vi "ivPIDantiWindup.vi"(4 "Saturation U":dbl, 6 "Saturation M":dbl, 7 "Reset":bool, 8 "PID Gains":cluster{"Kp":dbl, "Kd":dbl, "Ki":dbl, "Ts":dbl}={"Kp"=0.0, "Kd"=0.0, "Ki"=0.0, "Ts"=1.0}, 10 "Feedback":dbl, 11 "Reference":dbl) -> (3 "Control":dbl)   [LabVIEW 2016]
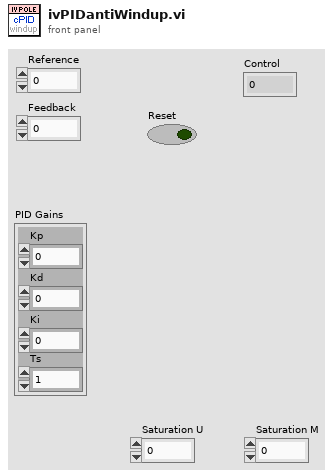
[diagram p1: front panel]
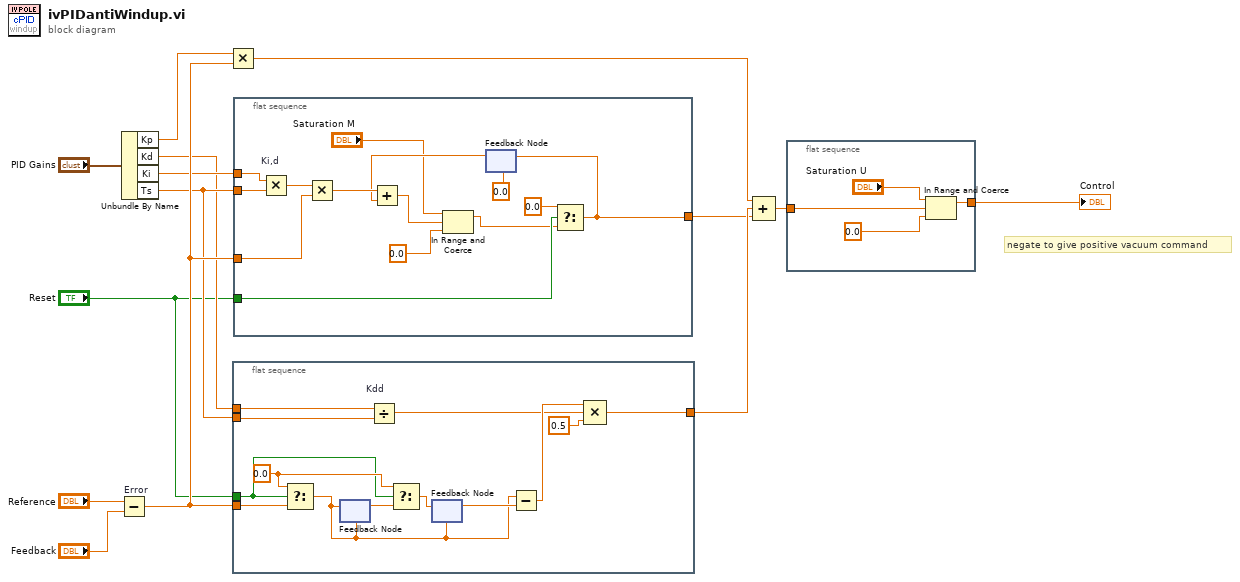
[diagram p0: block diagram]
diagram:
  # "negate to give positive vacuum command"
  n1 = Subtract "Error"(x="Reference", y="Feedback") -> (x-y=w7:dbl)
  n2 = Unbundle By Name("PID Gains") -> ("Kp"=w11:dbl, "Kd"=w4:dbl, "Ki"=w6:dbl, "Ts"=w5:dbl)
  n3 = Multiply(x=w11, y=w7) -> (x*y=w10:dbl)
  n4 = flat-sequence {
    tunnel: [w24] -> w9
    tunnel: w7 -> [w19]
    tunnel: w5 -> [w23]
    tunnel: w4 -> [w22]
    tunnel: "Reset" -> [w15]
    frame #0 {
      w16 = 0.0 ("t")
      n5 = Select(t=w16, s=w15, f=w19) -> (s? t:f=w20:dbl)
      n6 = feedback #1(w20) -> (w18:dbl)
      n7 = feedback-in #1(w20) -> ()
      n8 = Divide "Kdd"(x=w22, y=w23) -> (x/y=w21:dbl)
      n9 = Select(t=w16, s=w15, f=w18) -> (s? t:f=w17:dbl)
      n10 = feedback #2(w20) -> (w27:dbl)
      n11 = feedback-in #2(w17) -> ()
      n12 = Subtract(x=w20, y=w27) -> (x-y=w26:dbl)
      n13 = Compound Arithmetic op=MULTIPLY(w26, w21, 0.5 ("value")) -> (w24:dbl)
    }
  }
  n14 = flat-sequence {
    tunnel: [w30] -> w8
    tunnel: w7 -> [w41]
    tunnel: w6 -> [w39]
    tunnel: w5 -> [w37]
    tunnel: "Reset" -> [w33]
    frame #0 {
      n15 = Multiply "Ki,d"(x=w39, y=w37) -> (x*y=w38:dbl)
      n16 = Multiply(x=w38, y=w41) -> (x*y=w40:dbl)
      n17 = feedback #3(0.0 ("value")) -> (w34:dbl)
      n18 = Add(x=w40, y=w34) -> (x+y=w36:dbl)
      n19 = In Range and Coerce(upper limit="Saturation M", x=w36, lower limit=0.0 ("upper limit")) -> (coerced(x)=w32:dbl)  [unwired: 1 out]
      n20 = Select(t=0.0 ("value"), s=w33, f=w32) -> (s? t:f=w30:dbl)
      n21 = feedback-in #3(w30) -> ()
    }
  }
  n22 = Compound Arithmetic op=ADD(w10, w9, w8) -> (w3:dbl)
  n23 = flat-sequence {
    tunnel: w3 -> [w45]
    tunnel: [w44] -> w1
    frame #0 {
      n24 = In Range and Coerce(upper limit="Saturation U", x=w45, lower limit=0.0 ("upper limit")) -> (coerced(x)=w44:dbl)  [unwired: 1 out]
    }
  }
  "Control" <- w1
